vi "Start.vi"(8 "error in (no error)":errorcluster) -> (0 "error out":errorcluster, 3 "Engine":refnum<class "Engine.lvclass">)   [LabVIEW 2024, in "GLF.lvlib" / "Engine.lvclass"]
uses:
  Engine.lvclass
  Core.vi
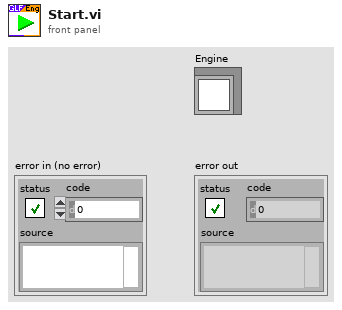
[diagram p1: front panel]
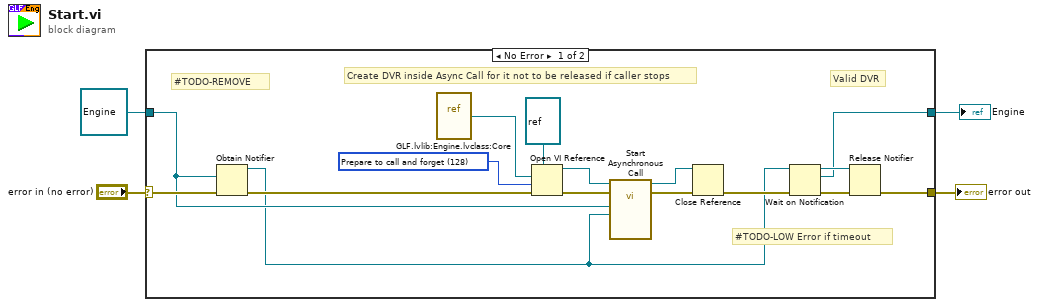
[diagram p0: block diagram]
diagram:
  n1 = case shown="No Error" "error in (no error)" {
    selector: "error in (no error)" -> [w14 w22]
    tunnel: [w8 w22] -> w3
    tunnel: refnum<class "Engine.lvclass"> refnum ("Engine in") -> [w6 w21]
    tunnel: [w7 w21] -> w1
    frame No Error {
      w12 = 128 items=["Record modifications"=1, "Open templates for editing"=2, "Prompt user to save"=4, "Prepare for reentrant run"=8, "Prompt to find missing subVIs"=16, "Hide loading dialog box"=32, "Enable simultaneous calls"=64, "Prepare to call and forget"=128, "Simultaneous call and forget"=192, "Prepare to call and collect"=256, "Simultaneous call and collect"=320]
      # "#TODO-REMOVE"
      # "#TODO-LOW Error if timeout"
      # "Valid DVR"
      # "Create DVR inside Async Call for it not to be released if caller stops"
      n2 = Obtain Notifier(notification data type=w6, error in (no error)=w14) -> (notifier out=w5:refnum<notifier>, error out=w13:errorcluster)  [unwired: 2 in, 1 out]
      n3 = vi-ref "GLF.lvlib:Engine.lvclass:Core.vi"() -> (w16:refnum<vi>)
      n4 = Open VI Reference(type specifier VI Refnum (for type only)=refnum<vi> refnum, vi path=w16, options=w12, error in (no error)=w13) -> (vi reference=w18:refnum<vi>, error out=w20:errorcluster)  [unwired: 2 in]
      n5 = call-by-ref "Start Asynchronous Call"(reference=w18, error in=w20, "Ready Notifier"=w5, "Engine in"=w6) -> (reference out=w17:refnum<vi>, error out=w19:errorcluster)  [unwired: 10 in]
      n6 = Close Reference(reference=w17, error in (no error)=w19) -> (error out=w11:errorcluster)
      n7 = Wait on Notification(notifier=w5, error in (no error)=w11) -> (notifier out=w9:refnum<notifier>, notification=w7:refnum<class "Engine.lvclass">, error out=w10:errorcluster)  [unwired: 2 in, 1 out]
      n8 = Release Notifier(notifier=w9, error in (no error)=w10) -> (error out=w8:errorcluster)  [unwired: 1 in, 2 out]
    }
    frame Error {
    }
  }
  "error out" <- w3
  "Engine" <- w1
